vi "Write_parameter.vi"(8 "error in (no error)":errorcluster caption="entrée d'erreur (pas d'erreur)", 10 "Parameter":string, 11 "Class Instrument Multimeter en entrée":refnum<class "Class Instrument Multimeter.lvclass">) -> (0 "error out":errorcluster caption="sortie d'erreur", 3 "Class Instrument Multimeter en sortie":refnum<class "Class Instrument Multimeter.lvclass">)   [LabVIEW 2020, in "Library Instrument & Equipement.lvlib" / "Library Instruments.lvlib" / "Class Instrument Multimeter.lvclass"]
uses:
  Class Instrument Multimeter.lvclass
  Commun VI/TypeDef/Command Multimeter/Parameter Multimeter.ctl
  Commun VI/TypeDef/Command Multimeter/Typedef Function.ctl
  Multimeter/Multimeter (Default)/Class Multimeter (Default).lvclass
  JSON API/JSON Value/Set from JSON string.vi
  Instrument (Default)/Class Instrument (Default).lvclass
  JSON API/JSON Value/JSON Value.lvclass
  Class Instrument Multimeter.lvclass/Class Instrument Multimeter.ctl
  JSON API/Variant JSON/Variant JSON.lvlib
  JSON API/Get Polymorphic/JSON GetSet.lvlib
  Commun VI/Library Commun.lvlib
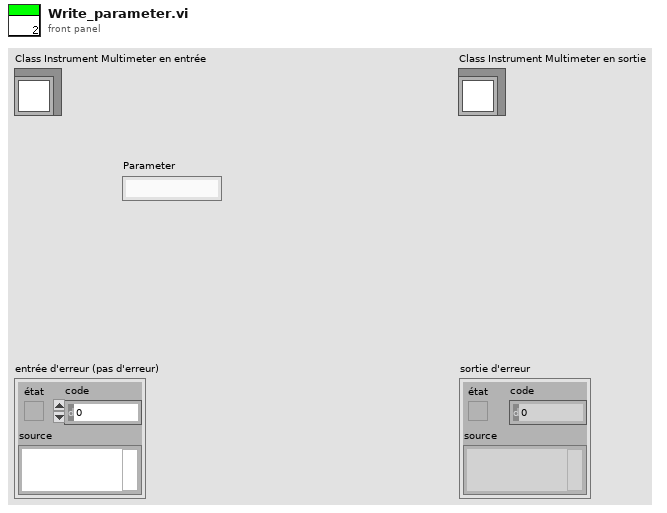
[diagram p1: front panel]
types:
  T1 = typedef "Library Commun.lvlib/Parameter Multimeter.ctl" = cluster{"Device @":refnum<visa-resource-name>, "Range":dbl, "Voltage Type":enum16{"AC", "DC"}, "Function":T2, "Class Multimeter":refnum<class "Class Multimeter (Default).lvclass">}
  T2 = typedef "Library Commun.lvlib/Typedef Function.ctl" = enum16{"Voltmeter", "Ammeter", "Continuity", "Ohmmeter", "Frequencymeter"}
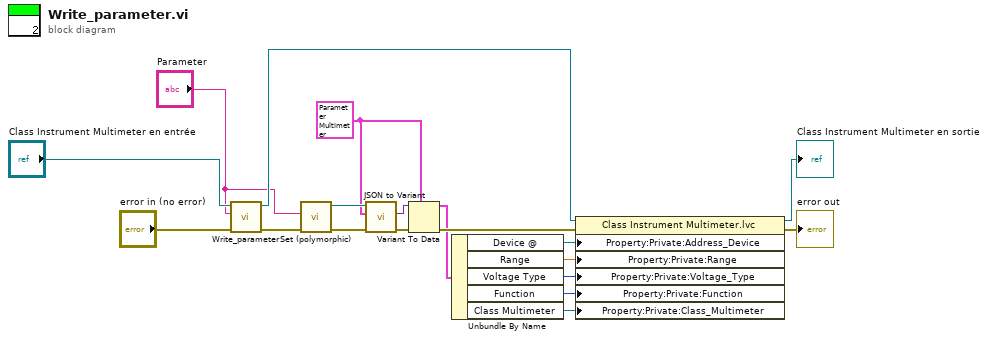
[diagram p0: block diagram]
diagram:
  w7 = T1 {"Device @"="", "Range"=0.0, "Voltage Type"=enum."AC", "Function"=enum."Voltmeter", "Class Multimeter"=refnum} ("Parameter")
  n1 = call-parent "Write_parameter.vi"("error in (no error)"="error in (no error)", "Parameter"="Parameter", "Class Instrument (Default) en entrée"="Class Instrument Multimeter en entrée") -> ("error out"=w4:errorcluster, "Class Instrument (Default) en sortie"=w3:refnum<class "Class Instrument Multimeter.lvclass">)  [unwired: 7 in]
  n2 = call-poly "Set (polymorphic).vi"("error in (no error)"=w4, "JSON stream"="Parameter") -> ("error out"=w17:errorcluster, "JSON Value out"=w19:refnum<class "JSON Value.lvclass">)  [unwired: 7 in, 1 out]
  n3 = call "JSON to Variant.vi"("error in (no error)"=w17, "Variant (Data Type)"=w7, "JSON Value"=w19) -> ("error out"=w18:errorcluster, "Variant out"=w16:variant)  [unwired: 7 in]
  n4 = Variant To Data(error in=w18, type=w7, Variant=w16) -> (data=w12:T1, error out=w13:errorcluster)
  n5 = Unbundle By Name(w12) -> ("Device @"=w8:refnum<visa-resource-name>, "Range"=w9:dbl, "Voltage Type"=w10:enum16{"AC", "DC"}, "Function"=w11:T2, "Class Multimeter"=w6:refnum<class "Class Multimeter (Default).lvclass">)
  n6 = property class="Class Instrument Multimeter.lvc"(reference=w3, error in=w13, "Property:Private:Address_Device"=w8, "Property:Private:Range"=w9, "Property:Private:Voltage_Type"=w10, "Property:Private:Function"=w11, "Property:Private:Class_Multimeter"=w6) -> (reference out=→"Class Instrument Multimeter en sortie":refnum<class "Class Instrument Multimeter.lvclass">, error out=→"error out":errorcluster)
